vi "DT_Merge.vi"(9 "Subset Triangles":cluster{"Triangles":i32[][]}[](array[cluster]), 10 "Subset":cluster{"start idx":i32, "length":i32}[](array[cluster]), 11 "Points In":cluster{"x":dbl, "y":dbl, "index":i32}[](array[cluster])) -> (0 "error":i32, 2 "Triangles":i32[][](array[numeric]), 3 "Points Out":cluster{"x":dbl, "y":dbl, "index":i32}[](array[cluster]))   [LabVIEW 2017, in "NI_AAL_Geometry.lvlib"]
uses:
  <vilib>/Analysis/NI_AAL_Geometry.lvlib
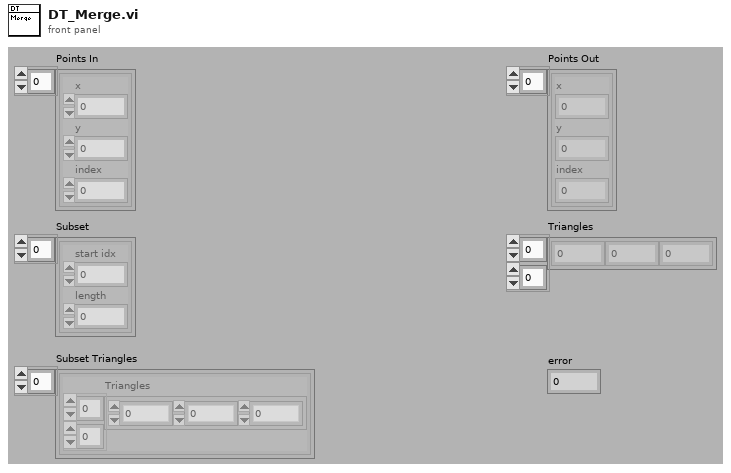
[diagram p1: front panel]
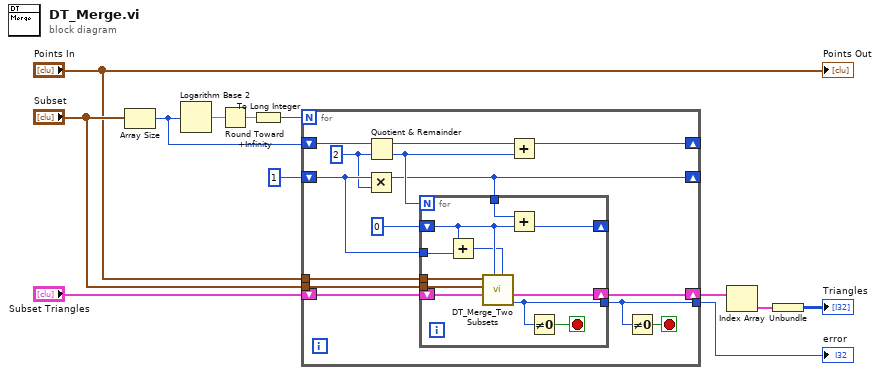
[diagram p0: block diagram]
diagram:
  n1 = Array Size(array="Subset") -> (size(s)=w12:i32)
  n2 = Logarithm Base 2(1:w12) -> (0:w8:dbl)
  n3 = Round Toward +Infinity(x=w8) -> (ceil(x): smallest int >= x=w7:dbl)
  n4 = To Long Integer(number=w7) -> (32bit integer=w5:i32)
  n5 = for {
    N: w5 -> [_]
    shift-right: [w20] -> _
    shift-left: 1 -> [w21]
    shift-right: [w24] -> _
    shift-left: w12 -> [w26]
    shift-right: [w17] -> w3
    shift-left: "Subset Triangles" -> [w18]
    tunnel: "Subset" -> [w16]
    tunnel: "Points In" -> [w19]
    tunnel: [w13] -> w1
    stop <- w14 stop-if-true
    w15 = 2 ("y")
    n6 = Multiply(x=w21, y=w15) -> (x*y=w20:i32)
    n7 = Quotient & Remainder(x=w26, y=w15) -> (x-y*floor(x/y)=w25:i32, floor(x/y)=w23:i32)
    n8 = for {
      N: w23 -> [_]
      shift-right: [w36] -> _
      shift-left: 0 -> [w34]
      tunnel: w20 -> [w37]
      tunnel: w21 -> [w35]
      shift-right: [w29] -> w17
      shift-left: w18 -> [w30]
      tunnel: w16 -> [w31]
      tunnel: w19 -> [w32]
      tunnel: [w27] -> w13
      stop <- w28 stop-if-true
      n9 = Add(x=w34, y=w35) -> (x+y=w33:i32)
      n10 = call <vilib>:"DT_Merge_Two Subsets.vi"("right subset"=w33, "left subset"=w34, "Subset Triangles In"=w30, "Subset"=w31, "Points In"=w32) -> ("error"=w27:i32, "Subset Triangles Out"=w29:cluster{"Triangles":i32[][]}[])  [unwired: 1 in, 4 out]
      n11 = Add(x=w37, y=w34) -> (x+y=w36:i32)
      n12 = Not Equal To 0?(x=w27) -> (x != 0?=w28:bool)
    }
    n13 = Add(x=w25, y=w23) -> (x+y=w24:i32)
    n14 = Not Equal To 0?(x=w13) -> (x != 0?=w14:bool)
  }
  "error" <- w1
  n15 = Index Array(array=w3) -> (element=w11:cluster{"Triangles":i32[][]})  [unwired: 1 in]
  n16 = Unbundle(w11) -> ("Triangles"=→"Triangles":i32[][])
  "Points Out" <- "Points In"
